vi "String Length.vi"() -> ()   [LabVIEW 2016]
panel:
  out "String Length":dbl
  in  "String":string
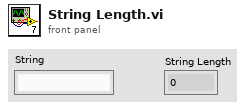
[diagram p1: front panel]
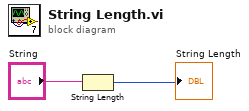
[diagram p0: block diagram]
diagram:
  n1 = String Length(string="String") -> (length=→"String Length":i32)
